vi "Transmit Message.vi"(6 "Response?":bool, 7 "Message":refnum<class "Message.lvclass">, 8 "error in (no error)":errorcluster, 9 "Requestee":string, 10 "Requestor":string, 11 "Mag Lab Measure Base in":refnum<class "Mag Lab Measure Base.lvclass">) -> (0 "error out":errorcluster, 3 "Mag Lab Measure Base out":refnum<class "Mag Lab Measure Base.lvclass">)   [LabVIEW 2015, in "Mag Lab Measure Base.lvclass"]
uses:
  Mag Lab Measure Base.lvclass
  <vilib>/ActorFramework/Message/Message.lvclass
  <vilib>/ActorFramework/Message Enqueuer/Message Enqueuer.lvclass/Message Enqueuer.ctl
  <vilib>/ActorFramework/Message Priority Queue/Priority Enqueue.vi
  <vilib>/ActorFramework/Message Enqueuer/Message Enqueuer.lvclass
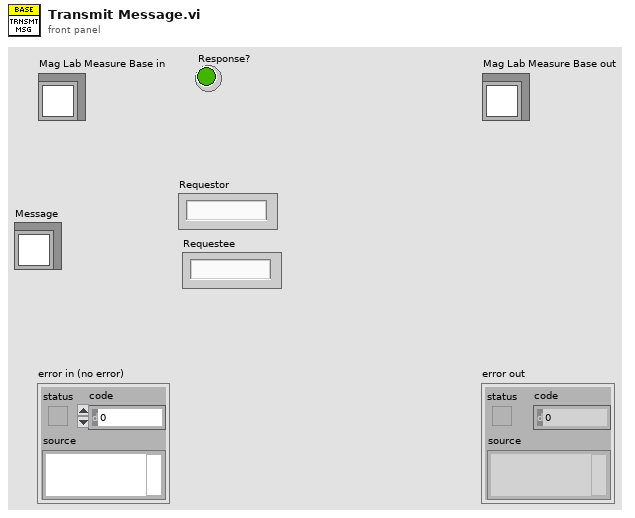
[diagram p1: front panel]
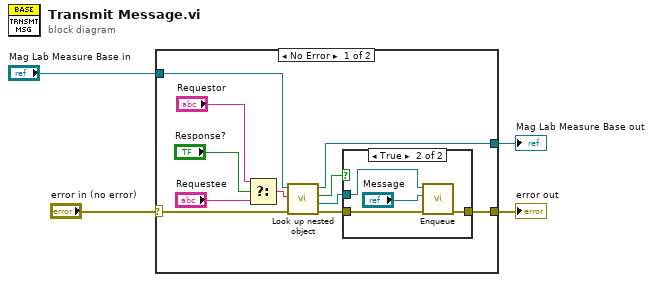
[diagram p0: block diagram]
diagram:
  n1 = case shown="No Error" "error in (no error)" {
    selector: "error in (no error)" -> [w5 w22]
    tunnel: [w9 w22] -> w3
    tunnel: [w10 w21] -> w1
    tunnel: "Mag Lab Measure Base in" -> [w15 w21]
    frame No Error {
      n2 = Select(t="Requestor", s="Response?", f="Requestee") -> (s? t:f=w14:string)
      n3 = call "Look up nested object.vi"("error in (no error)"=w5, "Object name"=w14, "Mag Lab Measure Base in"=w15) -> ("error out"=w11:errorcluster, "Object Queue"=w12:refnum<class "Message Enqueuer.lvclass">, "Found?"=w13:bool, "Mag Lab Measure Base out"=w10:refnum<class "Mag Lab Measure Base.lvclass">)  [unwired: 5 in]
      n4 = case shown="True" w13 {
        tunnel: w12 -> [_ w20]
        tunnel: w11 -> [w16 w19]
        tunnel: [w16 w18] -> w9
        frame False {
        }
        frame True {
          n5 = call <vilib>:"Enqueue.vi"("error in (no error)"=w19, "Message"="Message", "Message Enqueuer in"=w20) -> ("error out"=w18:errorcluster)  [unwired: 7 in, 1 out]
        }
      }
    }
    frame Error {
    }
  }
  "error out" <- w3
  "Mag Lab Measure Base out" <- w1
